vi "TIO Avg Field Data.vi"(8 "entrée d'erreur (pas d'erreur)":errorcluster, 10 "Component Index":i32, 11 "Tableau":T1(array[cluster])) -> (0 "sortie d'erreur":errorcluster, 1 "Z Average":dbl, 2 "Y Average":dbl, 3 "X Average":dbl, 4 "Total Average":dbl, 5 "dt":dbl, 7 "start":dbl)   [LabVIEW 2010]
panel:
  out "Total Data":dbl[](array[numeric])
  out "Z Data":dbl[](array[numeric])
  out "Y Data":dbl[](array[numeric])
  out "X Data":dbl[](array[numeric])
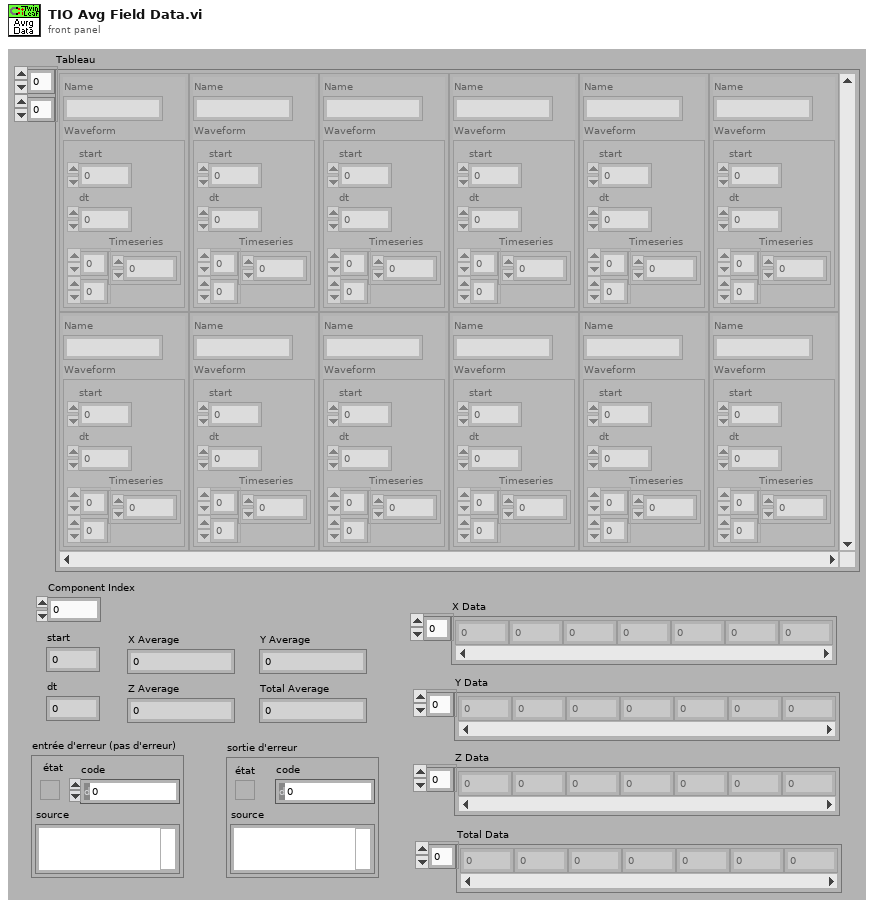
[diagram p1: front panel]
types:
  T1 = cluster{"Name":string, "Waveform":cluster{"start":dbl, "dt":dbl, "Timeseries":dbl[][]}}[][]
  T2 = cluster{"Name":string, "Waveform":cluster{"start":dbl, "dt":dbl, "Timeseries":dbl[][]}}
  T3 = cluster{"start":dbl, "dt":dbl, "Timeseries":dbl[][]}
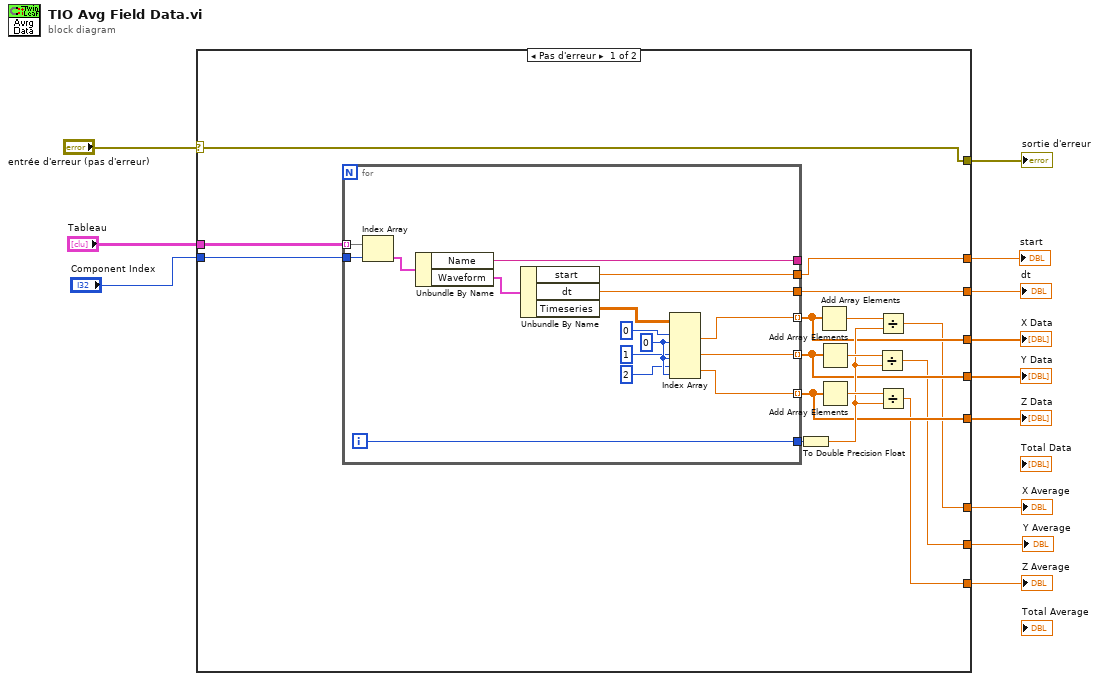
[diagram p0: block diagram]
diagram:
  n1 = case shown="Pas d'erreur" "entrée d'erreur (pas d'erreur)" {
    selector: "entrée d'erreur (pas d'erreur)" -> [w13 w45]
    tunnel: [w13 w45] -> w11
    tunnel: "Tableau" -> [w28 _]
    tunnel: "Component Index" -> [w27 _]
    tunnel: [w21 _] -> w8
    tunnel: [w20 _] -> w7
    tunnel: [w19 _] -> w6
    tunnel: [w18 _] -> w5
    tunnel: [w17 _] -> w4
    tunnel: [w16 _] -> w3
    tunnel: [w15 _] -> w2
    tunnel: [w14 _] -> w1
    frame No Error {
      n2 = for {
        tunnel: w28 -> [w44] mode=indexing
        tunnel: w27 -> [w42]
        tunnel: [w40] -> w21
        tunnel: [w39] -> w20
        tunnel: [w38] -> _
        tunnel: [w31] -> w19 mode=indexing
        tunnel: [w37] -> w25
        tunnel: [w30] -> w18 mode=indexing
        tunnel: [w29] -> w17 mode=indexing
        i -> [w37]
        w35 = 0 ("indice désactivé (col)")
        n3 = Index Array(array=w44, index=w42) -> (element=w43:T2)
        n4 = Unbundle By Name(w43) -> ("Name"=w38:string, "Waveform"=w41:T3)
        n5 = Unbundle By Name(w41) -> ("start"=w40:dbl, "dt"=w39:dbl, "Timeseries"=w36:dbl[][])
        n6 = Index Array(array=w36, index (row) #1=0 ("indice désactivé (ligne)"), index (col) #1=w35, index (row) #2=1 ("indice désactivé (ligne)"), index (col) #2=w35, index (row) #3=2 ("indice désactivé (ligne)"), index (col) #3=w35) -> (element #1=w31:dbl, element #2=w30:dbl, element #3=w29:dbl)
      }
      n7 = To Double Precision Float(number=w25) -> (double precision float=w22:dbl)
      n8 = Add Array Elements(numeric array=w19) -> (sum=w26:dbl)
      n9 = Add Array Elements(numeric array=w18) -> (sum=w24:dbl)
      n10 = Add Array Elements(numeric array=w17) -> (sum=w23:dbl)
      n11 = Divide(x=w24, y=w22) -> (x/y=w15:dbl)
      n12 = Divide(x=w26, y=w22) -> (x/y=w16:dbl)
      n13 = Divide(x=w23, y=w22) -> (x/y=w14:dbl)
    }
    frame Error {
    }
  }
  "sortie d'erreur" <- w11
  "start" <- w8
  "dt" <- w7
  "X Average" <- w3
  "X Data" <- w6
  "Z Data" <- w4
  "Z Average" <- w1
  "Y Data" <- w5
  "Y Average" <- w2
